vi "1D Fit Unscale Fit Outputs v3.vi"(0 "Fit Output in  (w sigma)":T5={"best nonlinear fit"=[], "best fit parameters"=[], "R^2"=0.0, "RMSE"=0.0, "error out"={"status"=FALSE, "code"=0, "source"=""}, "Fitting Method"=enum."Least Square", "number of function calls"=0, "number of iterations"=0, "covariance"=[], "Chi 2"=0.0, "DOF"=0, "Fit Convergence Criterion"=enum."Continue", "Fitting Algorithm"=enum."Levenberg-Marquardt", "Weighted Fit"=enum."Unweighted", "Gradient"=0.0, "|Delta Chi 2|"=0.0, "|Delta Chi 2|/Chi 2"=0.0, "Max |Delta a| /|a|"=0.0, "Lambda"=-1.0, "RSS"=0.0, "AIC"=0.0, "BIC"=0.0, "Max number of function calls"=0, "Max number of iterations"=0, "IRF"={"X Array"=[], "Y Array"=[]}, "IRF Normalization Factor"=0.0, "Decay Normalization Factor"=0.0, "Number of offset fits"=0, "Weighted Chi2"=-1.0, "Unweighted Chi2"=-1.0}, 1 "Fit Control Data in":T1, 5 "Decay Normalization Factor":dbl, 7 "IRF Normalization Factor":dbl, 9 "Scaled guess parameters (w tau)":dbl[](array[numeric]), 11 "Error In":errorcluster, 12 "# Points":i32, 13 "Order Lifetimes (F)":bool) -> (3 "Fit Control Data out (w sigma)":T1, 4 "Unscaled Fit Output out (w sigma)":T5={"best nonlinear fit"=[], "best fit parameters"=[], "R^2"=0.0, "RMSE"=0.0, "error out"={"status"=FALSE, "code"=0, "source"=""}, "Fitting Method"=enum."Least Square", "number of function calls"=0, "number of iterations"=0, "covariance"=[], "Chi 2"=0.0, "DOF"=0, "Fit Convergence Criterion"=enum."Continue", "Fitting Algorithm"=enum."Levenberg-Marquardt", "Weighted Fit"=enum."Unweighted", "Gradient"=0.0, "|Delta Chi 2|"=0.0, "|Delta Chi 2|/Chi 2"=0.0, "Max |Delta a| /|a|"=0.0, "Lambda"=-1.0, "RSS"=0.0, "AIC"=0.0, "BIC"=0.0, "Max number of function calls"=0, "Max number of iterations"=0, "IRF"={"X Array"=[], "Y Array"=[]}, "IRF Normalization Factor"=0.0, "Decay Normalization Factor"=0.0, "Number of offset fits"=0, "Weighted Chi2"=-1.0, "Unweighted Chi2"=-1.0}, 6 "Fitted unscaled parameters (w tau)":dbl[](array[numeric]), 8 "All unscaled parameters (w tau)":dbl[](array[numeric]), 10 "Unscaled guess parameters (w tau)":dbl[](array[numeric]), 15 "Error Out":errorcluster)   [LabVIEW 2021, in "Fits.lvlib"]
uses:
  Fits.lvlib
  Non-linear Fit Output v4.ctl
  Nonlinear Fit Method.ctl
  <vilib>/Analysis/Matrix/Datatypes/RealMatrix.ctl
  Convergence Criteria.ctl
  Non-linear Fitting Algorithm.ctl
  IRF(X)PSED/Fit Weights Type v2.ctl
  Graphs/XY Graph/XY Graph Plot Data.ctl
  Decay Convolution/Fit Control Data v2.ctl
  IRF(X)PSED/Decay Fit Parameters In List.ctl
  Decay Convolution/Decay Model.ctl
  <vilib>/Analysis/Matrix/NI_Matrix.lvlib
  Graphs/XY Graph/XY Graph Add-Ons.lvlib
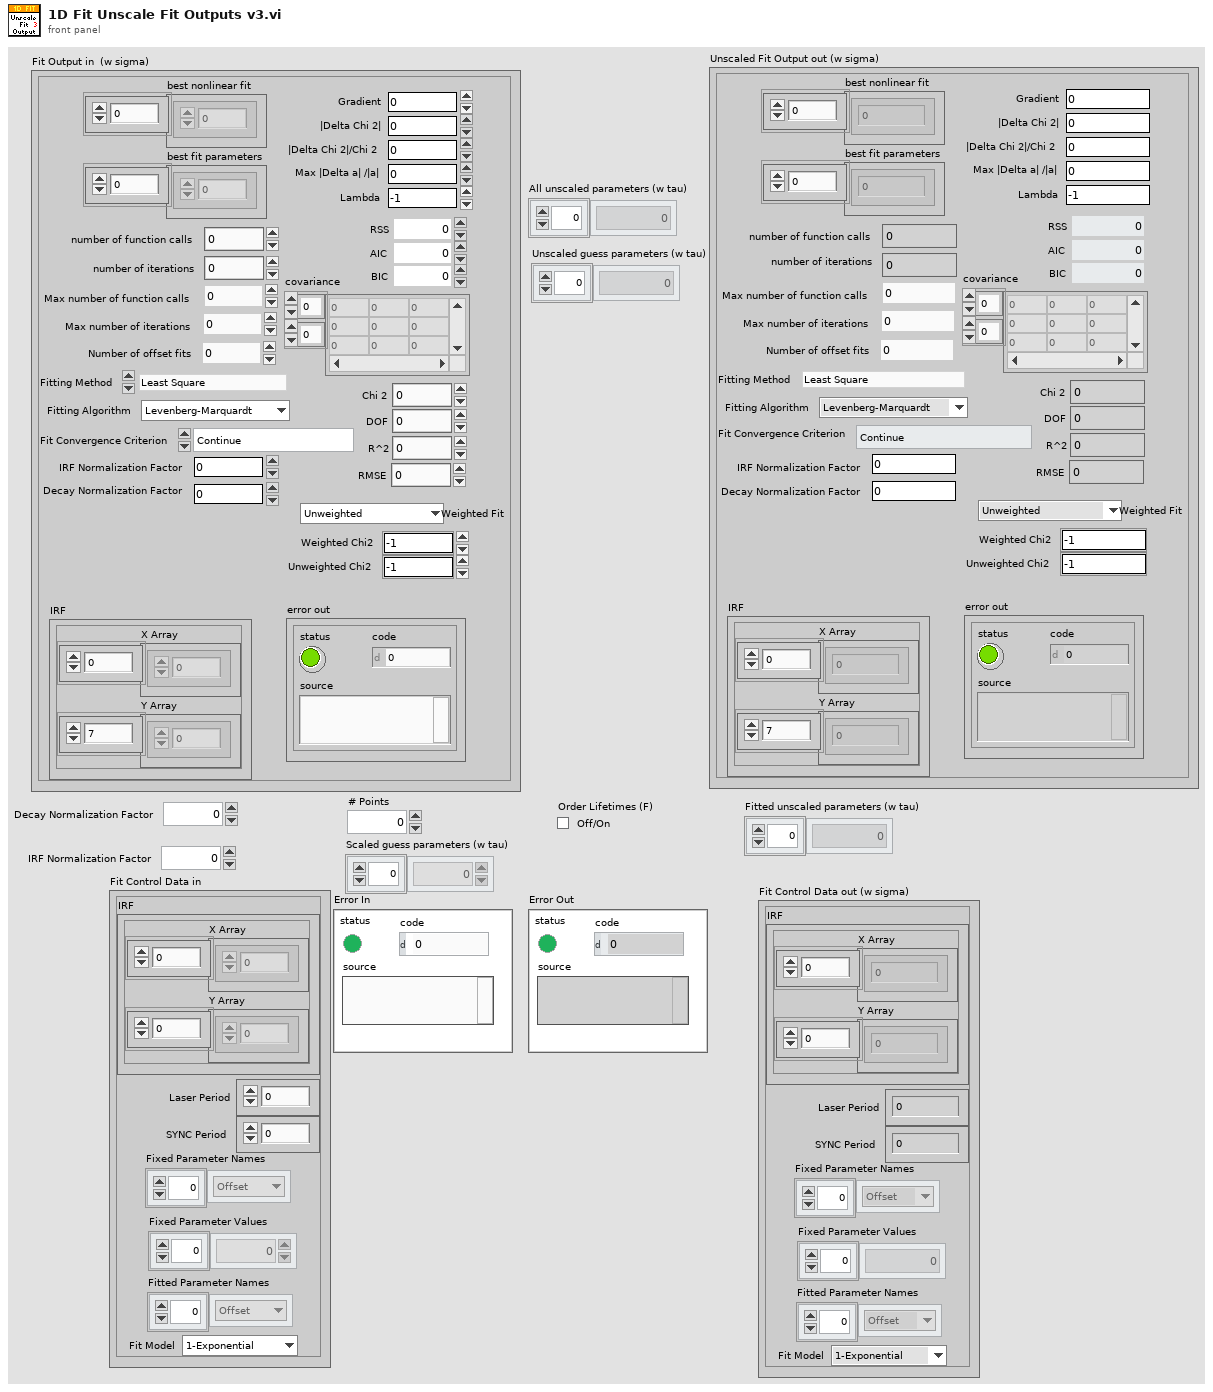
[diagram p1: front panel]
types:
  T1 = typedef "Fits.lvlib/Fit Control Data v2.ctl" = cluster{"IRF":T2, "Laser Period":dbl, "SYNC Period":dbl, "Fixed Parameter Names":T3[], "Fixed Parameter Values":dbl[], "Fitted Parameter Names":T3[], "Fit Model":T4}
  T2 = typedef "XY Graph Add-Ons.lvlib/XY Graph Plot Data.ctl" = cluster{"X Array":dbl[], "Y Array":dbl[]}
  T3 = typedef "Fits.lvlib/Decay Fit Parameters In List.ctl" = enum16{"Offset", "Baseline", "A_1", "tau_1", "A_2", "tau_2"}
  T4 = typedef "Fits.lvlib/Decay Model.ctl" = enum16{"1-Exponential", "2-Exponentials"}
  T5 = typedef "Fits.lvlib/Non-linear Fit Output v4.ctl" = cluster{"best nonlinear fit":dbl[], "best fit parameters":dbl[], "R^2":dbl, "RMSE":dbl, "error out":errorcluster, "Fitting Method":T6, "number of function calls":i32, "number of iterations":i32, "covariance":T7, "Chi 2":dbl, "DOF":i32, "Fit Convergence Criterion":T8, "Fitting Algorithm":T9, "Weighted Fit":T10, "Gradient":dbl, "|Delta Chi 2|":dbl, "|Delta Chi 2|/Chi 2":dbl, "Max |Delta a| /|a|":dbl, "Lambda":dbl, "RSS":dbl, "AIC":dbl, "BIC":dbl, "Max number of function calls":i32, "Max number of iterations":i32, "IRF":T2, "IRF Normalization Factor":dbl, "Decay Normalization Factor":dbl, "Number of offset fits":i32, "Weighted Chi2":dbl, "Unweighted Chi2":dbl}
  T6 = typedef "Fits.lvlib/Nonlinear Fit Method.ctl" = enum16{"Least Square", "Least Absolute Residual", "Bisquare", "MLE"}
  T7 = typedef "NI_Matrix.lvlib/RealMatrix.ctl" = dbl[][]
  T8 = typedef "Fits.lvlib/Convergence Criteria.ctl" = enum16{"Continue", "Tolerances Exceeded", "Max Time Exceeded", "Max Iterations Exceeded", "Max Function Evaluations Exceeded", "Scale Range Exceeded"}
  T9 = typedef "Fits.lvlib/Non-linear Fitting Algorithm.ctl" = enum16{"Levenberg-Marquardt", "Trust-Region Dogleg"}
  T10 = typedef "Fits.lvlib/Fit Weights Type v2.ctl" = enum16{"Unweighted", "1/Variance (Neyman)", "1/Variance (Pearson)", "Best of All"}
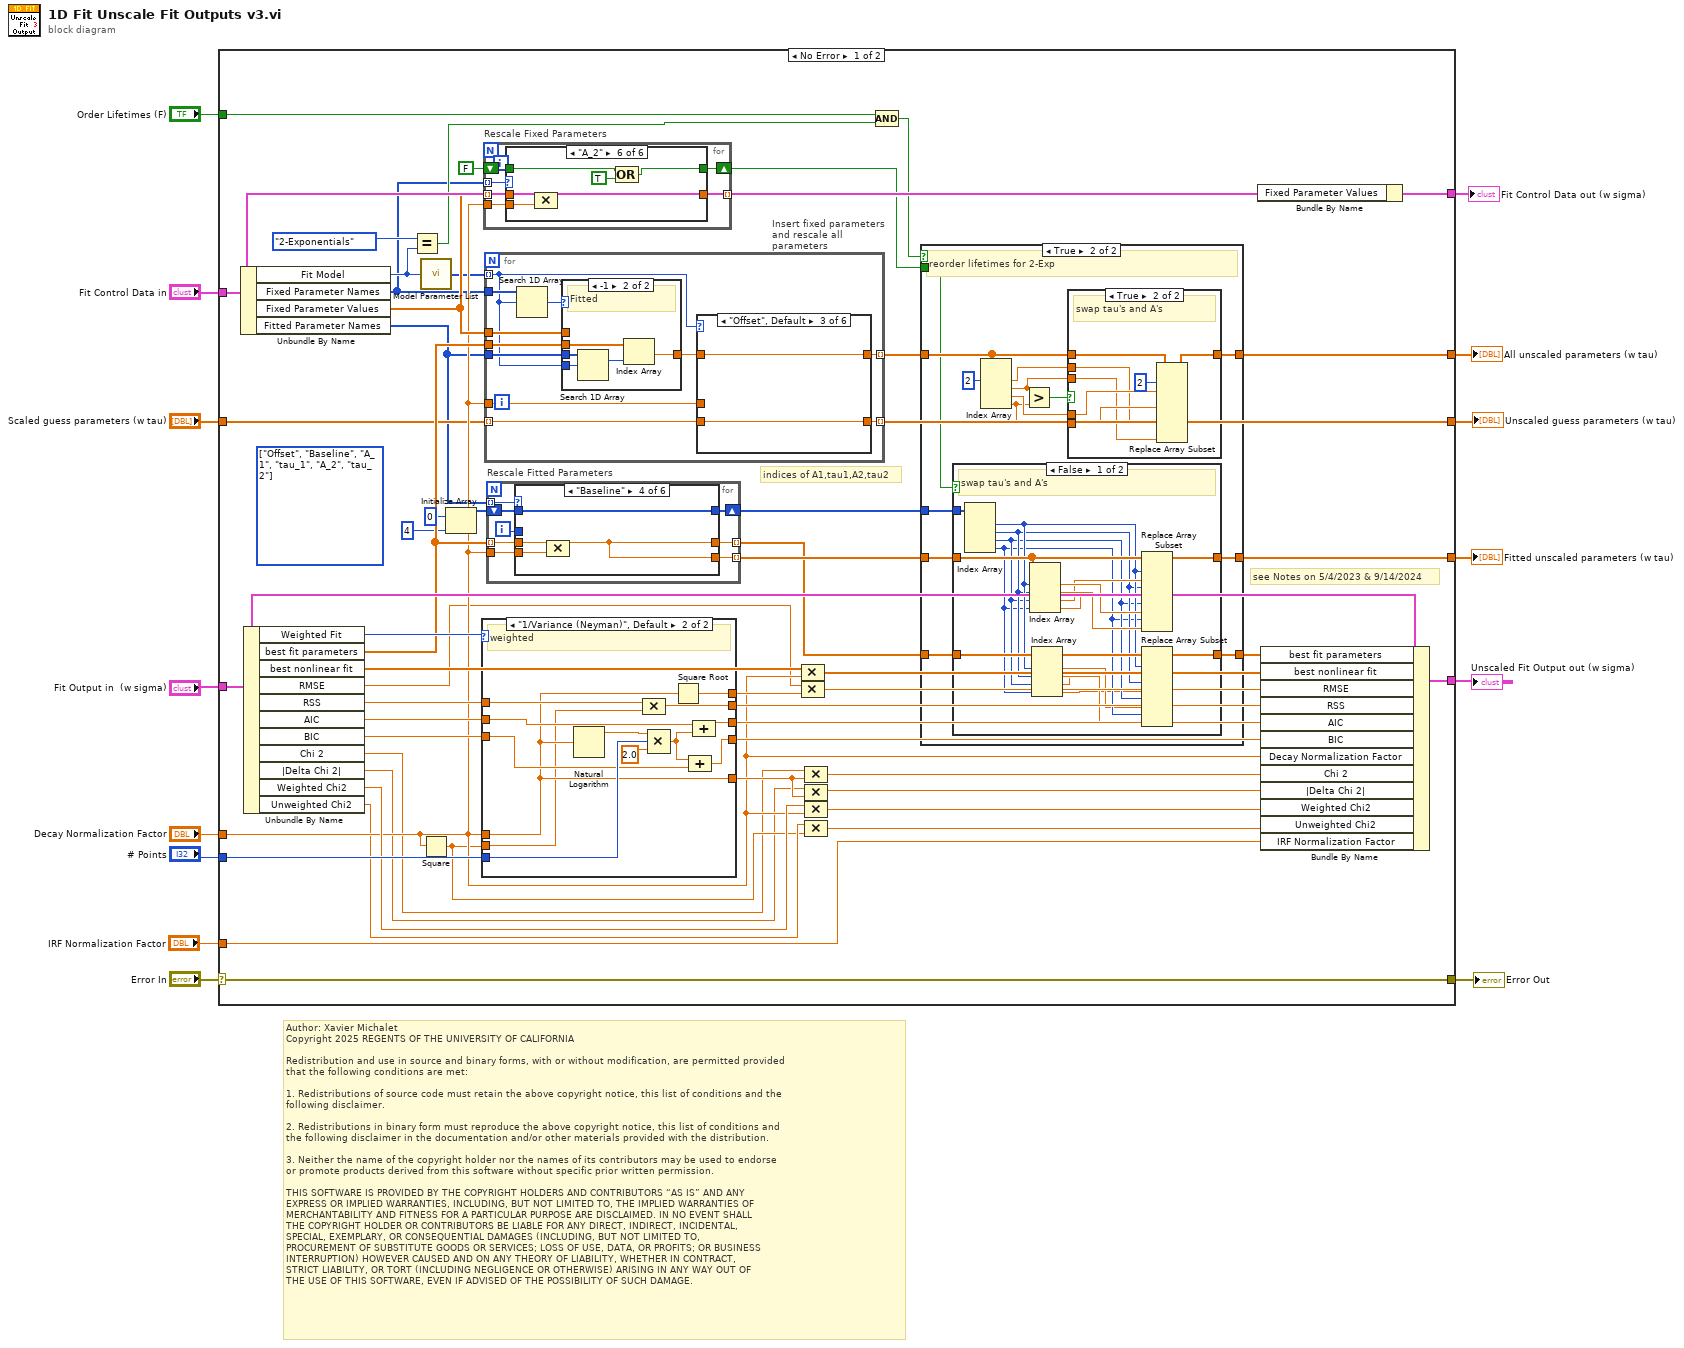
[diagram p0: block diagram]
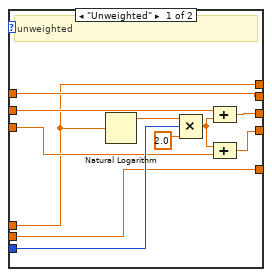
[diagram p5: hidden frame]
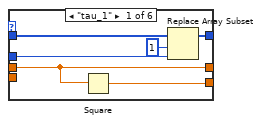
[diagram p6: hidden frame]
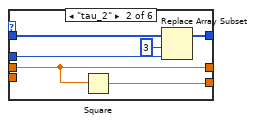
[diagram p7: hidden frame]
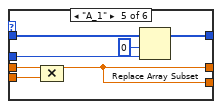
[diagram p9: hidden frame]
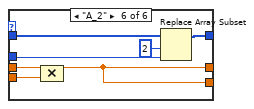
[diagram p10: hidden frame]
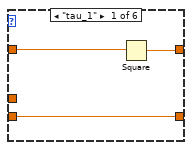
[diagram p11: hidden frame]
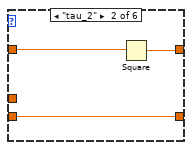
[diagram p12: hidden frame]
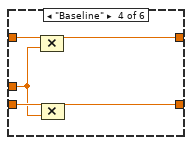
[diagram p13: hidden frame]
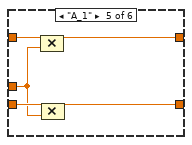
[diagram p14: hidden frame]
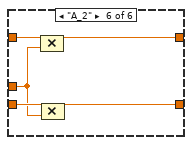
[diagram p15: hidden frame]
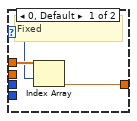
[diagram p16: hidden frame]
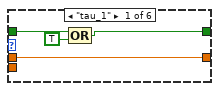
[diagram p17: hidden frame]
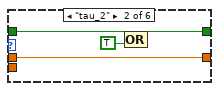
[diagram p18: hidden frame]
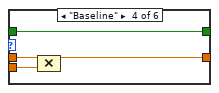
[diagram p20: hidden frame]
diagram:
  # "Author: Xavier Michalet\nCopyright 2025 REGENTS OF THE UNIVERSITY OF CALIFORNIA\n\nRedistribution and use in source and binary forms, with or without modification, are permitted provided\nthat the following conditions are met:\n\n1. Redistributions of source code must retain the above copyright notice, this list of conditions and the\nfollowing disclaimer.\n\n2. Redistributions in binary form must reproduce the above copyright notice, this list of conditions and\nthe following disclaimer in the documentation and/or other materials provided with the distribution.\n\n3. Neither the name of the copyright holder nor the names of its contributors may be used to endorse \nor promote products derived from this software without specific prior written permission.\n\nTHIS SOFTWARE IS PROVIDED BY THE COPYRIGHT HOLDERS AND CONTRIBUTORS “AS IS” AND ANY \nEXPRESS OR IMPLIED WARRANTIES, INCLUDING, BUT NOT LIMITED TO, THE IMPLIED WARRANTIES OF\nMERCHANTABILITY AND FITNESS FOR A PARTICULAR PURPOSE ARE DISCLAIMED. IN NO EVENT SHALL\nTHE COPYRIGHT HOLDER OR CONTRIBUTORS BE LIABLE FOR ANY DIRECT, INDIRECT, INCIDENTAL, \nSPECIAL, EXEMPLARY, OR CONSEQUENTIAL DAMAGES (INCLUDING, BUT NOT LIMITED TO, \nPROCUREMENT OF SUBSTITUTE GOODS OR SERVICES; LOSS OF USE, DATA, OR PROFITS; OR BUSINESS\nINTERRUPTION) HOWEVER CAUSED AND ON ANY THEORY OF LIABILITY, WHETHER IN CONTRACT, \nSTRICT LIABILITY, OR TORT (INCLUDING NEGLIGENCE OR OTHERWISE) ARISING IN ANY WAY OUT OF\nTHE USE OF THIS SOFTWARE, EVEN IF ADVISED OF THE POSSIBILITY OF SUCH DAMAGE."
  n1 = case shown="No Error" "Error In" {
    selector: "Error In" -> [w62 w253]
    tunnel: "Fit Output in  (w sigma)" -> [w69 _]
    tunnel: [w68 _] -> w13
    tunnel: "Fit Control Data in" -> [w60 w252]
    tunnel: [w27 _] -> w12
    tunnel: "IRF Normalization Factor" -> [w38 _]
    tunnel: "Decay Normalization Factor" -> [w46 _]
    tunnel: [w62 w253] -> w9
    tunnel: [w58 w252] -> w8
    tunnel: [w24 _] -> w5
    tunnel: "# Points" -> [w57 _]
    tunnel: "Scaled guess parameters (w tau)" -> [w37 _]
    tunnel: [w22 _] -> w2
    tunnel: "Order Lifetimes (F)" -> [w35 _]
    frame No Error {
      (unwired) T3[] [enum."Offset", enum."Baseline", enum."A_1", enum."tau_1", enum."A_2", enum."tau_2"] items=["Offset", "Baseline", "A_1", "tau_1", "A_2", "tau_2"] ("Fitted Parameter Names")
      # "indices of A1,tau1,A2,tau2"
      # "see Notes on 5/4/2023 & 9/14/2024"
      n2 = Unbundle By Name(w60) -> ("Fit Model"=w33:T4, "Fixed Parameter Names"=w30:T3[], "Fixed Parameter Values"=w59:dbl[], "Fitted Parameter Names"=w19:T3[])
      n3 = Unbundle By Name(w69) -> ("Weighted Fit"=w63:T10, "best fit parameters"=w61:dbl[], "best nonlinear fit"=w67:dbl[], "RMSE"=w41:dbl, "RSS"=w56:dbl, "AIC"=w55:dbl, "BIC"=w54:dbl, "Chi 2"=w39:dbl, "|Delta Chi 2|"=w40:dbl, "Weighted Chi2"=w47:dbl, "Unweighted Chi2"=w45:dbl)
      n4 = Equal?(x=Decay_Model."2-Exponentials" ("Fit Model"), y=w33) -> (x = y?=w32:bool)
      n5 = call "Model Parameter List.vi"("Fit Model"=w33) -> ("Model Parameter List"=w28:T3[])
      n6 = Square(x=w46) -> (x^2=w44:dbl)
      n7 = Initialize Array(0 ("element"), 4 ("dimension size")) -> (w18:i32[])
      n8 = case shown="\"1/Variance (Neyman)\", Default" w63 {
        tunnel: w46 -> [w115 w126]
        tunnel: [w115 w137] -> w64
        tunnel: w57 -> [w118 w133]
        tunnel: w56 -> [w121 w131]
        tunnel: w55 -> [w120 w130]
        tunnel: w54 -> [w117 w128]
        tunnel: [w121 w132] -> w53
        tunnel: [w119 w129] -> w52
        tunnel: [w116 w127] -> w51
        tunnel: [w114 w126] -> w49
        tunnel: w44 -> [w114 w125]
        frame "Unweighted" {
          # "unweighted"
          n9 = Natural Logarithm(1:w115) -> (0:w124:dbl)
          n10 = Compound Arithmetic op=MULTIPLY(w124, w118, 2.0 ("value")) -> (w122:dbl)
          n11 = Compound Arithmetic op=ADD(w120, w122) -> (w119:dbl)
          n12 = Compound Arithmetic op=ADD(w122, w117) -> (w116:dbl)
        }
        frame "1/Variance (Neyman)", Default {
          # "weighted"
          n13 = Natural Logarithm(1:w126) -> (0:w136:dbl)
          n14 = Compound Arithmetic op=MULTIPLY(w131, w125) -> (w132:dbl)
          n15 = Compound Arithmetic op=MULTIPLY(w136, w133, 2.0 ("value")) -> (w134:dbl)
          n16 = Square Root(x=w126) -> (sqrt(x)=w137:dbl)
          n17 = Compound Arithmetic op=ADD(w134, w128) -> (w127:dbl)
          n18 = Compound Arithmetic op=ADD(w130, w134) -> (w129:dbl)
        }
      }
      n19 = for "Rescale Fixed Parameters" {
        tunnel: w30 -> [w225] mode=indexing
        tunnel: w59 -> [w224] mode=indexing
        tunnel: w46 -> [w223]
        tunnel: [w222] -> w31 mode=indexing
        shift-right: [w220] -> w20
        shift-left: FALSE -> [w221]
        n20 = case shown="\"A_2\"" w225 {
          tunnel: w224 -> [w229 w233 w235 w239 w245 w251]
          tunnel: w223 -> [_ _ _ w238 w244 w250]
          tunnel: [w229 w233 w235 w237 w243 w249] -> w222
          tunnel: w221 -> [w228 w232 w234 w236 w242 w248]
          tunnel: [w226 w230 w234 w236 w240 w246] -> w220
          frame "tau_1" {
            n21 = Compound Arithmetic op=OR(w228, TRUE ("value")) -> (w226:bool)
          }
          frame "tau_2" {
            n22 = Compound Arithmetic op=OR(w232, TRUE ("value")) -> (w230:bool)
          }
          frame "Offset", Default {
          }
          frame "Baseline" {
            n23 = Compound Arithmetic op=MULTIPLY(w239, w238) -> (w237:dbl)
          }
          frame "A_1" {
            n24 = Compound Arithmetic op=MULTIPLY(w245, w244) -> (w243:dbl)
            n25 = Compound Arithmetic op=OR(w242, TRUE ("value")) -> (w240:bool)
          }
          frame "A_2" {
            n26 = Compound Arithmetic op=MULTIPLY(w251, w250) -> (w249:dbl)
            n27 = Compound Arithmetic op=OR(w248, TRUE ("value")) -> (w246:bool)
          }
        }
      }
      n28 = for "Insert fixed parameters and rescale all parameters" {
        tunnel: w28 -> [w181] mode=indexing
        tunnel: w30 -> [w188]
        tunnel: w46 -> [w184]
        tunnel: w19 -> [w182]
        tunnel: w59 -> [w183]
        tunnel: w61 -> [w186]
        tunnel: [w180] -> w29 mode=indexing
        tunnel: w37 -> [w179] mode=indexing
        tunnel: [w178] -> w22 mode=indexing
        n29 = Search 1D Array(1D array=w188, element=w181) -> (index of element=w187:i32)  [unwired: 1 in]
        n30 = case shown="-1" w187 {
          selector: w187 -> [w213 _]
          tunnel: w186 -> [_ w217]
          tunnel: [w212 w215] -> w185
          tunnel: w183 -> [w214 _]
          tunnel: w182 -> [_ w219]
          tunnel: w181 -> [_ w218]
          frame 0, Default {
            # "Fixed"
            n31 = Index Array(array=w214, index=w213) -> (element=w212:dbl)
          }
          frame -1 {
            # "Fitted"
            n32 = Search 1D Array(1D array=w219, element=w218) -> (index of element=w216:i32)  [unwired: 1 in]
            n33 = Index Array(array=w217, index=w216) -> (element=w215:dbl)
          }
        }
        n34 = case shown="\"Offset\", Default" w181 {
          tunnel: w185 -> [w191 w194 w196 w201 w206 w211]
          tunnel: w184 -> [_ _ _ w198 w203 w208]
          tunnel: [w190 w193 w196 w200 w205 w210] -> w180
          tunnel: w179 -> [w189 w192 w195 w199 w204 w209]
          tunnel: [w189 w192 w195 w197 w202 w207] -> w178
          frame "tau_1" {
            n35 = Square(x=w191) -> (x^2=w190:dbl)
          }
          frame "tau_2" {
            n36 = Square(x=w194) -> (x^2=w193:dbl)
          }
          frame "Offset", Default {
          }
          frame "Baseline" {
            n37 = Compound Arithmetic op=MULTIPLY(w201, w198) -> (w200:dbl)
            n38 = Compound Arithmetic op=MULTIPLY(w199, w198) -> (w197:dbl)
          }
          frame "A_1" {
            n39 = Compound Arithmetic op=MULTIPLY(w206, w203) -> (w205:dbl)
            n40 = Compound Arithmetic op=MULTIPLY(w204, w203) -> (w202:dbl)
          }
          frame "A_2" {
            n41 = Compound Arithmetic op=MULTIPLY(w211, w208) -> (w210:dbl)
            n42 = Compound Arithmetic op=MULTIPLY(w209, w208) -> (w207:dbl)
          }
        }
      }
      n43 = for "Rescale Fitted Parameters" {
        tunnel: w19 -> [w145] mode=indexing
        tunnel: w61 -> [w144] mode=indexing
        tunnel: w46 -> [w143]
        tunnel: [w142] -> w25 mode=indexing
        tunnel: [w141] -> w26 mode=indexing
        shift-right: [w139] -> w15
        shift-left: w18 -> [w140]
        i -> [w138]
        n44 = case shown="\"Baseline\"" w145 {
          tunnel: w144 -> [w151 w157 w159 w162 w169 w176]
          tunnel: w143 -> [_ _ _ w163 w170 w177]
          tunnel: [w151 w157 w159 w161 w168 w175] -> w142
          tunnel: [w150 w156 w159 w161 w168 w175] -> w141
          tunnel: w140 -> [w147 w154 w158 w160 w167 w173]
          tunnel: [w148 w153 w158 w160 w166 w172] -> w139
          tunnel: w138 -> [w146 w152 _ _ w164 w171]
          frame "tau_1" {
            n45 = Square(x=w151) -> (x^2=w150:dbl)
            n46 = Replace Array Subset(array=w147, new element=w146, index=1) -> (w148:i32[])
          }
          frame "tau_2" {
            n47 = Square(x=w157) -> (x^2=w156:dbl)
            n48 = Replace Array Subset(array=w154, new element=w152, index=3) -> (w153:i32[])
          }
          frame "Offset", Default {
          }
          frame "Baseline" {
            n49 = Compound Arithmetic op=MULTIPLY(w162, w163) -> (w161:dbl)
          }
          frame "A_1" {
            n50 = Compound Arithmetic op=MULTIPLY(w169, w170) -> (w168:dbl)
            n51 = Replace Array Subset(array=w167, new element=w164, index=0) -> (w166:i32[])
          }
          frame "A_2" {
            n52 = Compound Arithmetic op=MULTIPLY(w176, w177) -> (w175:dbl)
            n53 = Replace Array Subset(array=w173, new element=w171, index=2) -> (w172:i32[])
          }
        }
      }
      n54 = Compound Arithmetic op=MULTIPLY(w67, w46) -> (w66:dbl[])
      n55 = Compound Arithmetic op=MULTIPLY(w41, w64) -> (w65:dbl)
      n56 = Compound Arithmetic op=MULTIPLY(w39, w49) -> (w50:dbl)
      n57 = Compound Arithmetic op=MULTIPLY(w40, w49) -> (w48:dbl)
      n58 = Compound Arithmetic op=MULTIPLY(w47, w46) -> (w43:dbl)
      n59 = Compound Arithmetic op=MULTIPLY(w45, w44) -> (w42:dbl)
      n60 = Compound Arithmetic op=AND(w35, w32) -> (w36:bool)
      n61 = case shown="True" w36 {
        tunnel: w29 -> [w72 w85]
        tunnel: [w72 w80] -> w27
        tunnel: w26 -> [w71 w76]
        tunnel: w25 -> [w70 w75]
        tunnel: [w71 w74] -> w24
        tunnel: [w70 w73] -> w23
        tunnel: w20 -> [_ w78]
        tunnel: w15 -> [_ w77]
        frame False {
          # "Do not reorder lifetimes"
        }
        frame True {
          # "reorder lifetimes for 2-Exp"
          n62 = case shown="False" w78 {
            tunnel: w77 -> [w103 _]
            tunnel: w76 -> [w101 w105]
            tunnel: w75 -> [w95 w104]
            tunnel: [w102 w105] -> w74
            tunnel: [w96 w104] -> w73
            frame False {
              # "swap tau's and A's"
              n63 = Index Array(array=w103) -> (element #1=w94:i32, element #2=w93:i32, element #3=w92:i32, element #4=w91:i32)  [unwired: 4 in]
              n64 = Index Array(array=w101, index #1=w94, index #2=w93, index #3=w92, index #4=w91) -> (element #1=w100:dbl, element #2=w99:dbl, element #3=w98:dbl, element #4=w97:dbl)
              n65 = Index Array(array=w95, index #1=w94, index #2=w93, index #3=w92, index #4=w91) -> (element #1=w90:dbl, element #2=w89:dbl, element #3=w88:dbl, element #4=w87:dbl)
              n66 = Replace Array Subset(array=w101, new element #1=w98, index #1=w94, new element #2=w97, index #2=w93, new element #3=w100, index #3=w92, new element #4=w99, index #4=w91) -> (w102:dbl[])
              n67 = Replace Array Subset(array=w95, new element #1=w88, index #1=w94, new element #2=w87, index #2=w93, new element #3=w90, index #3=w92, new element #4=w89, index #4=w91) -> (w96:dbl[])
            }
            frame True {
              # "one of the A's or tau's is fixed"
            }
          }
          n68 = Index Array(array=w85, index #1=2 ("index")) -> (element #1=w84:dbl, element #2=w81:dbl, element #3=w83:dbl, element #4=w82:dbl)  [unwired: 3 in]
          n69 = Greater?(x=w81, y=w82) -> (0:w86:bool)
          n70 = case shown="True" w86 {
            tunnel: w85 -> [w106 w113]
            tunnel: w84 -> [_ w108]
            tunnel: w83 -> [_ w110]
            tunnel: w82 -> [_ w109]
            tunnel: w81 -> [_ w107]
            tunnel: [w106 w112] -> w80
            frame False {
              # "No swapping needed"
            }
            frame True {
              # "swap tau's and A's"
              n71 = Replace Array Subset(array=w113, new element #1=w110, index #1=2 ("index"), new element #2=w109, new element #3=w108, new element #4=w107) -> (w112:dbl[])  [unwired: 3 in]
            }
          }
        }
      }
      n72 = Bundle By Name(cluster=w60, "Fixed Parameter Values"=w31) -> (w58:T1)
      n73 = Bundle By Name(cluster=w69, "best fit parameters"=w23, "best nonlinear fit"=w66, "RMSE"=w65, "RSS"=w53, "AIC"=w52, "BIC"=w51, "Decay Normalization Factor"=w46, "Chi 2"=w50, "|Delta Chi 2|"=w48, "Weighted Chi2"=w43, "Unweighted Chi2"=w42, "IRF Normalization Factor"=w38) -> (w68:T5)
    }
    frame Error {
    }
  }
  "Unscaled Fit Output out (w sigma)" <- w13
  "All unscaled parameters (w tau)" <- w12
  "Error Out" <- w9
  "Fit Control Data out (w sigma)" <- w8
  "Fitted unscaled parameters (w tau)" <- w5
  "Unscaled guess parameters (w tau)" <- w2
